vi "Build Numeric Table.vi"(0 "report in":refnum<class "NI_report.lvclass">, 1 "column headers":string[](array[string]), 2 "rows/page":i32, 5 "row headers":string[](array[string]), 9 "numerical data":dbl[][](array[numeric]) format="%.2f", 11 "error in (no error)":errorcluster, 12 "format string (%.2f)":string, 13 "nonzero rows/page":bool) -> (4 "report out":refnum<class "NI_report.lvclass">, 15 "error out":errorcluster)   [LabVIEW 2017, in "NI_ReportGenerationCore.lvlib"]
uses:
  <vilib>/Utility/NIReport.llb/NI_ReportGenerationCore.lvlib
  <vilib>/Utility/NIReport.llb/NI_report.lvclass
  <vilib>/Utility/NIReport.llb/Append Report Text (str wrap).vi
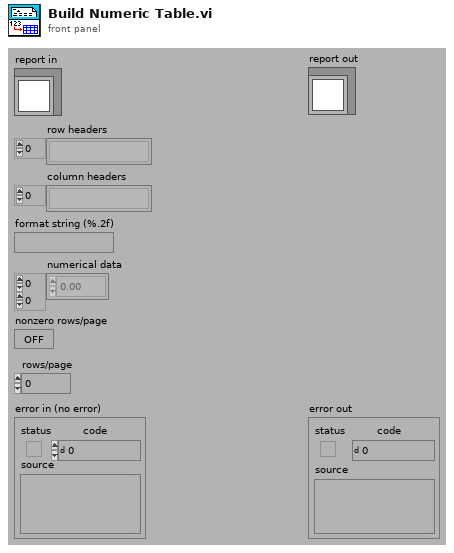
[diagram p1: front panel]
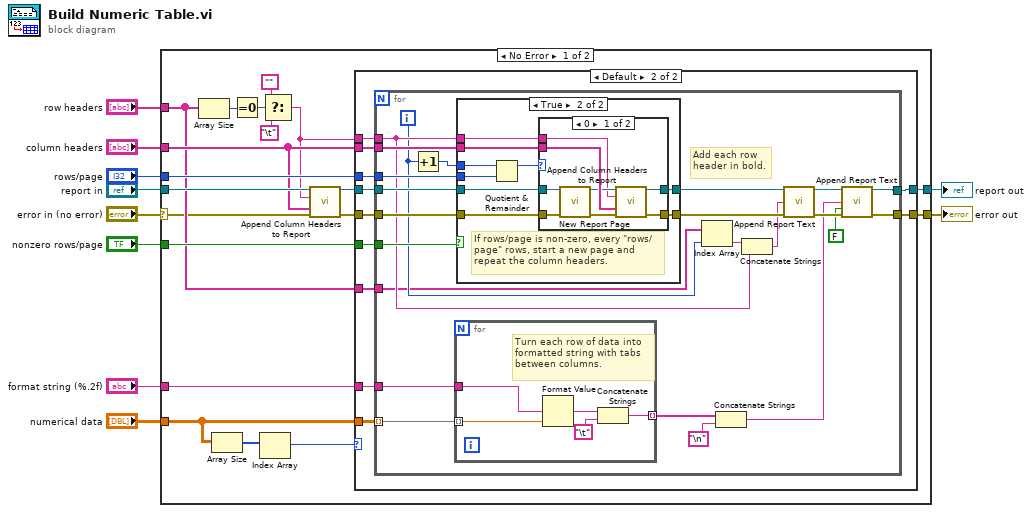
[diagram p0: block diagram]
diagram:
  n1 = case shown="No Error" "error in (no error)" {
    selector: "error in (no error)" -> [w12 w92]
    tunnel: "report in" -> [w25 w93]
    tunnel: "rows/page" -> [w23 _]
    tunnel: "nonzero rows/page" -> [w22 _]
    tunnel: "format string (%.2f)" -> [w21 _]
    tunnel: [w20 w93] -> w6
    tunnel: [w19 w92] -> w5
    tunnel: "column headers" -> [w17 _]
    tunnel: "row headers" -> [w16 _]
    tunnel: "numerical data" -> [w13 _]
    frame No Error {
      n2 = Array Size(array=w16) -> (size(s)=w29:i32)
      n3 = Array Size(array=w13) -> (size(s)=w14:i32[])
      n4 = Equal To 0?(x=w29) -> (x = 0?=w28:bool)
      n5 = Index Array(array=w14) -> (element=w11:i32)  [unwired: 1 in]
      n6 = Select(t="", s=w28, f="\t") -> (s? t:f=w15:string)
      n7 = call <vilib>:"Append Column Headers to Report.vi"("report in"=w25, "initial header"=w15, "column headers"=w17, "error in (no error)"=w12) -> ("report out"=w24:refnum<class "NI_report.lvclass">, "error out"=w18:errorcluster)  [unwired: 10 in]
      n8 = case shown="Default" w11 {
        tunnel: w15 -> [_ w42]
        tunnel: w17 -> [_ w41]
        tunnel: w24 -> [w31 w40]
        tunnel: w18 -> [w30 w39]
        tunnel: w23 -> [_ w38]
        tunnel: w22 -> [_ w37]
        tunnel: w16 -> [_ w36]
        tunnel: w13 -> [_ w35]
        tunnel: w21 -> [_ w34]
        tunnel: [w31 w33] -> w20
        tunnel: [w30 w32] -> w19
        frame 0 {
        }
        frame Default {
          n9 = for {
            tunnel: w42 -> [w58]
            tunnel: w41 -> [w65]
            tunnel: w40 -> [w63]
            tunnel: w39 -> [w62]
            tunnel: w38 -> [w61]
            tunnel: w37 -> [w60]
            tunnel: w36 -> [w56]
            tunnel: w35 -> [w55] mode=indexing
            tunnel: w34 -> [w54]
            tunnel: [w44] -> w33
            tunnel: [w43] -> w32
            i -> [w57]
            # "Add each row\nheader in bold."
            n10 = Increment(x=w57) -> (x+1=w64:i32)
            n11 = for {
              tunnel: w54 -> [w70]
              tunnel: w55 -> [w67] mode=indexing
              tunnel: [w66] -> w52 mode=indexing
              # "Turn each row of data into\nformatted string with tabs\nbetween columns."
              n12 = Format Value(format string=w70, value (0)=w67) -> (output string=w69:string)  [unwired: 1 in]
              n13 = Concatenate Strings(w69, "\t") -> (w66:string)
            }
            n14 = case shown="True" w60 {
              tunnel: w64 -> [_ w81]
              tunnel: w61 -> [_ w80]
              tunnel: w62 -> [w71 w78]
              tunnel: [w71 w77] -> w50
              tunnel: w63 -> [w72 w76]
              tunnel: [w72 w75] -> w51
              tunnel: w58 -> [_ w74]
              tunnel: w65 -> [_ w79]
              frame False {
              }
              frame True {
                # "If rows/page is non-zero, every \"rows/page\" rows, start a new page and repeat the column headers."
                n15 = Quotient & Remainder(x=w81, y=w80) -> (x-y*floor(x/y)=w73:i32)  [unwired: 1 out]
                n16 = case shown="0" w73 {
                  tunnel: w79 -> [w89 _]
                  tunnel: w74 -> [w82 _]
                  tunnel: w78 -> [w88 w90]
                  tunnel: [w86 w90] -> w77
                  tunnel: w76 -> [w85 w91]
                  tunnel: [w84 w91] -> w75
                  frame 0 {
                    n17 = call-dynamic "New Report Page.vi"("report in"=w85, "error in (no error)"=w88) -> ("report out"=w83:refnum<class "NI_report.lvclass">, "error out"=w87:errorcluster)  [unwired: 12 in]
                    n18 = call <vilib>:"Append Column Headers to Report.vi"("report in"=w83, "initial header"=w82, "column headers"=w89, "error in (no error)"=w87) -> ("report out"=w84:refnum<class "NI_report.lvclass">, "error out"=w86:errorcluster)  [unwired: 10 in]
                  }
                  frame Default {
                  }
                }
              }
            }
            n19 = Index Array(array=w56, index=w57) -> (element=w59:string)
            n20 = Concatenate Strings(w52, "\n") -> (w47:string)
            n21 = Concatenate Strings(w59, w58) -> (w45:string)
            n22 = call-poly <vilib>:"Append Report Text.vi"("report in"=w51, "text"=w45, "error in (no error)"=w50) -> ("report out"=w49:refnum<class "NI_report.lvclass">, "error out"=w48:errorcluster)  [unwired: 9 in, 2 out]
            n23 = call-poly <vilib>:"Append Report Text.vi"("report in"=w49, "text"=w47, "append on new line? (F)"=FALSE ("append newline? (F)"), "error in (no error)"=w48) -> ("report out"=w44:refnum<class "NI_report.lvclass">, "error out"=w43:errorcluster)  [unwired: 8 in, 2 out]
          }
        }
      }
    }
    frame Error {
    }
  }
  "error out" <- w5
  "report out" <- w6
